vi "process_main.vi"(7 "FGV_mods":enum16{"Init", "Exec", "End"}(ring)=enum."Exec", 8 "Error In":errorcluster, 11 "DataIn":variant) -> (0 "Error Out":errorcluster, 3 "DataOut":variant)   [LabVIEW 2016]
uses:
  process_data.ctl
  MainFGV/MainFGV_data.ctl
  MainFGV/Settings/config_board.ctl
  MainFGV/MainFGV_mods.ctl
  Log/log_mods.ctl
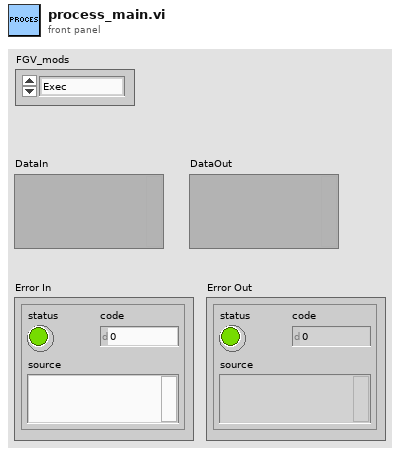
[diagram p1: front panel]
types:
  T1 = typedef "MainFGV_data.ctl" = cluster{"TestDir":path, "TestName":string, "Simulation":bool, "task":refnum<k21>, "data_file":refnum<file>, "burts_file":refnum<file>, "log_file":refnum<file>, "Rate":dbl, "SamplesPerChannel":dbl, "AcqQueue":refnum<queue>, "StartTime":timestamp, "config_channels":T2[], "DAQmx Device":tag}
  T2 = typedef "config_board.ctl" = cluster{"Sens0":dbl, "Active0":bool, "Sens1":dbl, "Active1":bool, "Sens2":dbl, "Active2":bool, "Sens3":dbl, "Active3":bool}
  T3 = typedef "process_data.ctl" = cluster{"AcqQueue":refnum<queue>, "rate":dbl}
  T4 = typedef "log_mods.ctl" = enum16{"Init", "LogFileRefnum", "SetStatus", "WriteAcel", "WriteToLog", "End"}
  T5 = typedef "MainFGV_mods.ctl" = enum16{"Init", "Config", "CreateTask", "Register", "Acquire", "Start", "Burst", "Record", "End"}
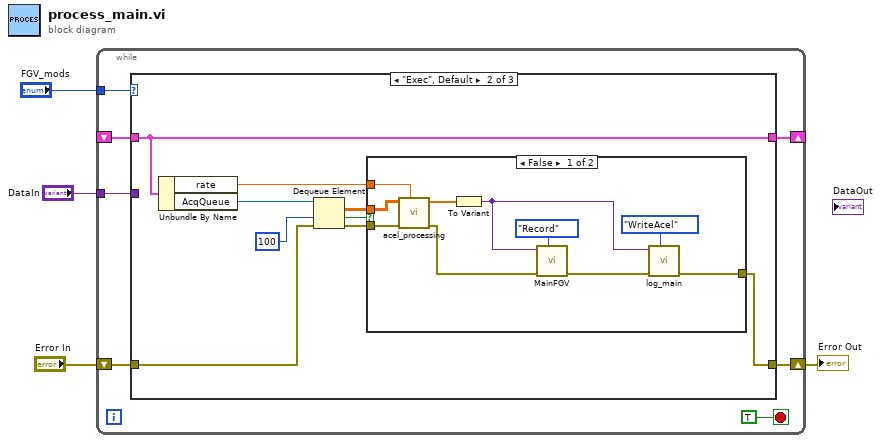
[diagram p0: block diagram]
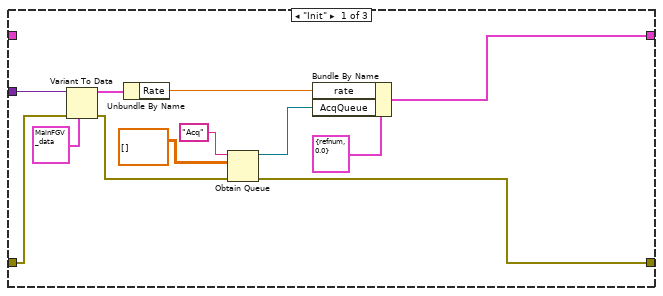
[diagram p2: hidden frame]
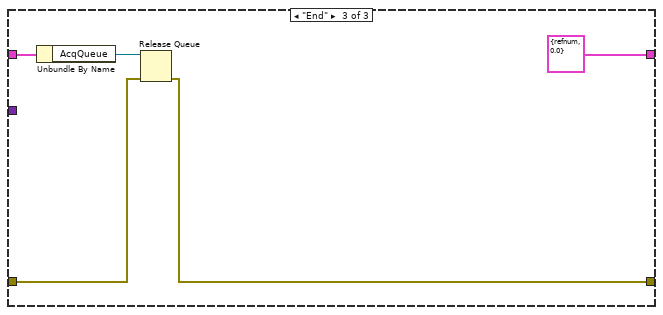
[diagram p4: hidden frame]
diagram:
  n1 = while {
    tunnel: "DataIn" -> [w10]
    tunnel: "FGV_mods" -> [w9]
    shift-right: [w8] -> _
    shift-left: _ -> [w7]
    shift-right: [w5] -> w1
    shift-left: "Error In" -> [w6]
    stop <- TRUE stop-if-true
    n2 = case shown="\"Exec\", Default" w9 {
      tunnel: w10 -> [w23 _ _]
      tunnel: [w19 w32 T3 {"AcqQueue"=refnum, "rate"=0.0} ("process_data")] -> w8
      tunnel: w7 -> [_ w32 w48]
      tunnel: w6 -> [w22 w29 w45]
      tunnel: [w14 w25 w44] -> w5
      frame "Init" {
        n3 = Variant To Data(error in=w22, type=T1 {"TestDir"=path "", "TestName"="", "Simulation"=FALSE, "task"="", "data_file"=refnum, "burts_file"=refnum, "log_file"=refnum, "Rate"=0.0, "SamplesPerChannel"=0.0, "AcqQueue"=refnum, "StartTime"=timestamp(0 s since 1904-01-01), "config_channels"=[], "DAQmx Device"=""} ("MainFGV_data"), Variant=w23) -> (data=w13:T1, error out=w18:errorcluster)
        n4 = Unbundle By Name(w13) -> ("Rate"=w12:dbl)
        n5 = Obtain Queue(name (unnamed)="Acq", element data type=dbl[][] [] ("2D array"), error in (no error)=w18) -> (queue out=w15:refnum<queue>, error out=w14:errorcluster)  [unwired: 2 in, 1 out]
        n6 = Bundle By Name(cluster=T3 {"AcqQueue"=refnum, "rate"=0.0} ("process_data"), "rate"=w12, "AcqQueue"=w15) -> (w19:T3)
      }
      frame "Exec", Default {
        n7 = Unbundle By Name(w32) -> ("rate"=w24:dbl, "AcqQueue"=w31:refnum<queue>)
        n8 = Dequeue Element(queue=w31, timeout in ms (-1)=100, error in (no error)=w29) -> (element=w30:dbl[][], timed out?=w27:bool, error out=w26:errorcluster)  [unwired: 1 out]
        n9 = case shown="False" w27 {
          tunnel: w30 -> [w38 _]
          tunnel: w26 -> [w36 w43]
          tunnel: [w42 w43] -> w25
          tunnel: w24 -> [w37 _]
          frame False {
            n10 = call "acel_processing.vi"("rate"=w37, "error in"=w36, "acelData"=w38) -> ("error out"=w33:errorcluster, "RMS"=w35:dbl[])  [unwired: 7 in]
            n11 = To Variant(anything=w35) -> (Variant=w34:variant)
            n12 = call "MainFGV.vi"("FGV_mods"=MainFGV_mods."Record", "Error In"=w33, "DataIn"=w34) -> ("Error Out"=w39:errorcluster)  [unwired: 7 in, 1 out]
            n13 = call "log_main.vi"("FGV_mods"=log_mods."WriteAcel", "Error In"=w39, "DataIn"=w34) -> ("Error Out"=w42:errorcluster)  [unwired: 7 in, 1 out]
          }
          frame True {
          }
        }
      }
      frame "End" {
        n14 = Unbundle By Name(w48) -> ("AcqQueue"=w47:refnum<queue>)
        n15 = Release Queue(queue=w47, error in (no error)=w45) -> (error out=w44:errorcluster)  [unwired: 1 in, 2 out]
      }
    }
  }
  "Error Out" <- w1
